vi "Bertta_v04.vi"() -> ()   [LabVIEW 2015]
uses:
  BERTTA.dll
panel:
  in  "Tab Control":T1(tab)
  in  "Description":string
  in  "Project name":string
  in  "User (initials)":string
  out "Mettler":dynamicdata(graph)
  out "?":dynamicdata(graph)
  in  "Balances":bool[](array[boolean])
  out "Waveform Chart 3":dynamicdata(graph)
  out "Table":string[][](table)
  in  "Headers":string[](array[string])
  in  "Seq":dbl[][](array[numeric])=[[20.0, 60.0, 40.0], [60.0, 40.0, 20.0], [100.0, 100.0, 100.0]]
  out "Waveform Chart":dynamicdata(graph)
  in  "PAUSE":bool
  in  "START SEQUENCE":bool
  out "setpoint":dbl
  out "Tcurrent":dbl
  in  "Step":i32
  out "Tinit":dbl
  out "Tset":dbl
  out "Ramp time":dbl
  in  "Heidolph":dbl(slide) scale=0.0..1000.0
  in  "Ismatec":dbl(slide) scale=0.0..160.0
  in  "?":T2(tab)
  out "rc":i32
  in  "Device port":dbl=1.0
  out "Debug msg":dbl
  in  "Device port":dbl=20.0
  in  "Device port":i32=2
  out "Weight":dbl
  out "Weight":dbl
  in  "Device port":i32=6
  in  "Device port":i32=15
  # "1"
  # "2"
  # "3"
  # "4"
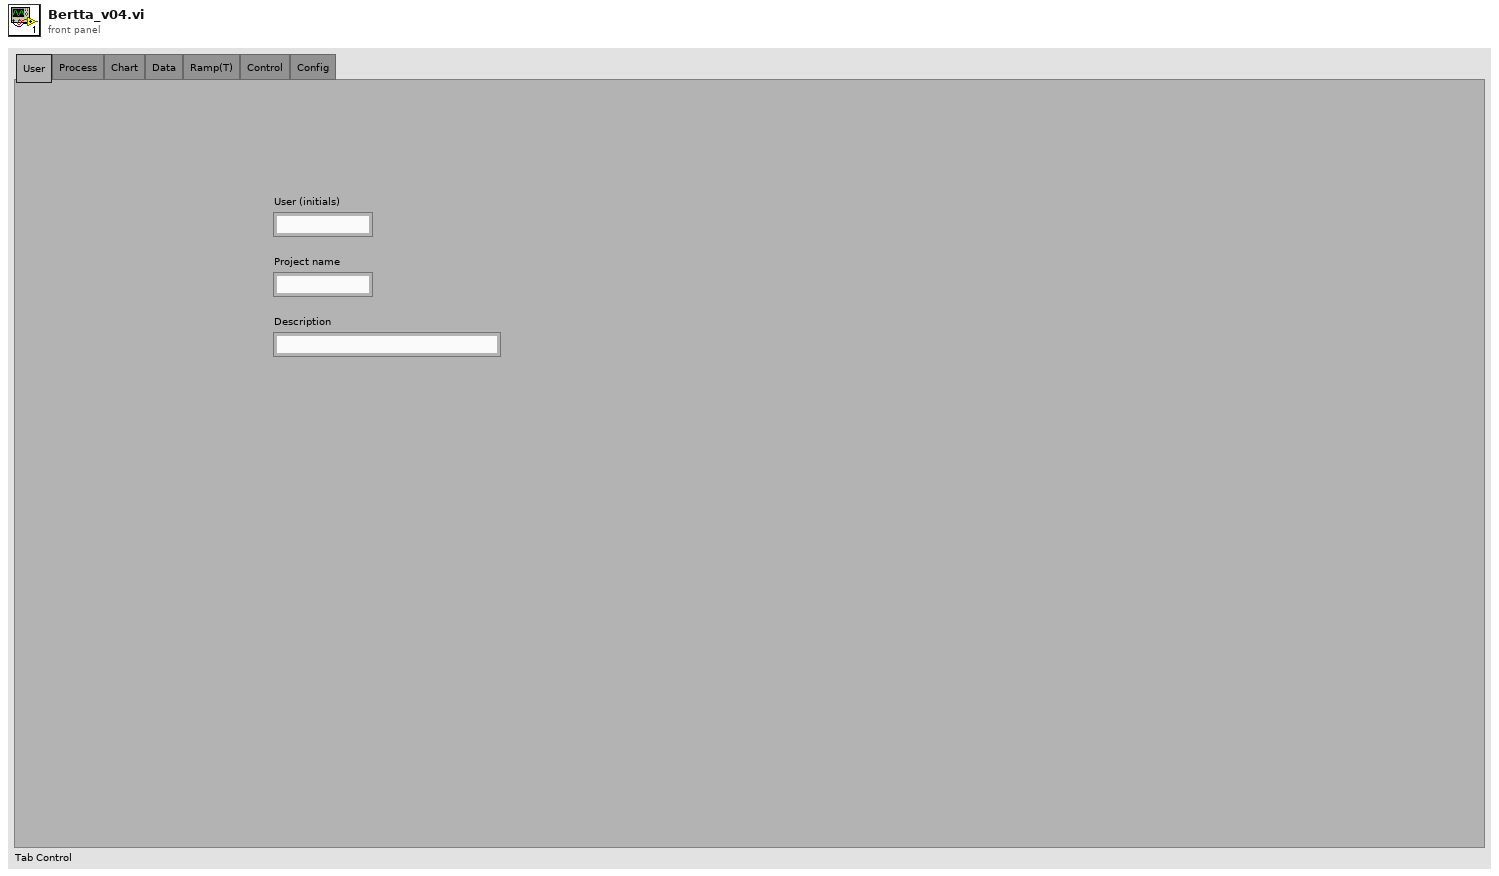
[diagram p1: front panel]
types:
  T1 = enum32{"User", "Process", "Chart", "Data", "Ramp(T)", "Control", "Config"}
  T2 = enum32{"DB / File", "Lauda", "Heidolph", "Mettler 1", "Mettler 2", "Mettler 3", "Ismatec 1"}
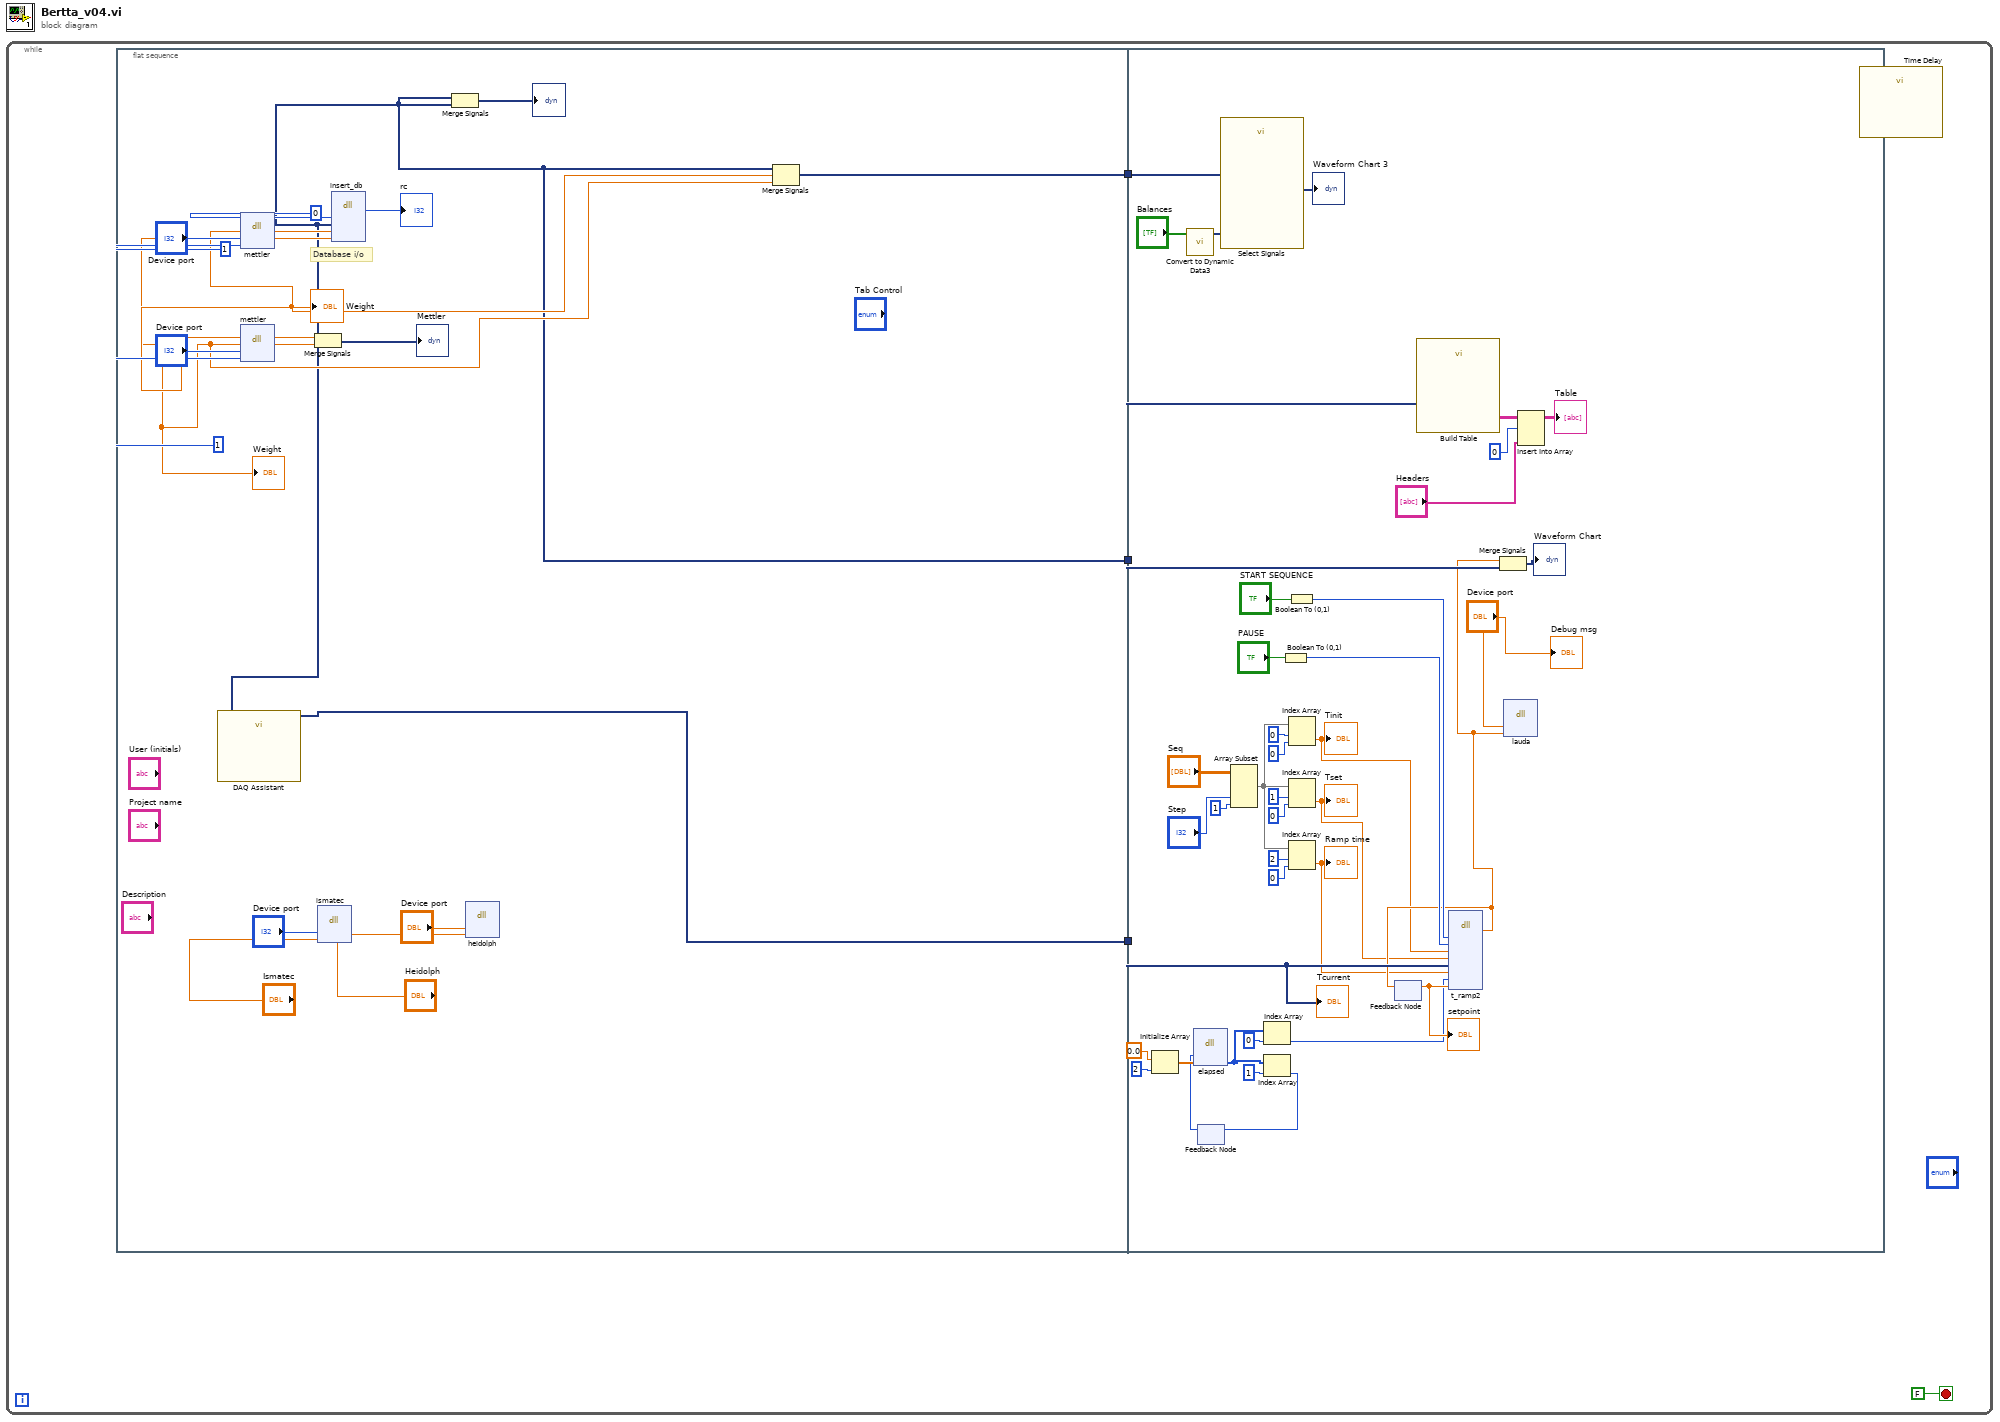
[diagram p0: block diagram]
diagram:
  n1 = while {
    stop <- FALSE stop-if-true
    n2 = flat-sequence {
      tunnel: [w6] -> w3
      tunnel: [w5] -> w2
      tunnel: [w5] -> w1
      tunnel: w3 -> [w53]
      tunnel: w2 -> [w42]
      tunnel: w1 -> [w35]
      frame #0 {
        # "Database i/o"
        n3 = call "DAQ Assistant"() -> ("data"=w5:dynamicdata)  [unwired: 17 in, 2 out]
        n4 = dll-call lib="C:/Users/xlaraser/Documents/Visual Studio 2017/Projects/Bertta/BERTTA/Debug/BERTTA.dll" fn="mettler"("port"="Device port", "msg"=1) -> ("return type"=w8:dbl)  [unwired: 5 in, 2 out]
        "Weight" <- w8
        n5 = dll-call lib="C:/Users/xlaraser/Documents/Visual Studio 2017/Projects/Bertta/BERTTA/Debug/BERTTA.dll" fn="mettler"("port"="Device port", "msg"=1) -> ("return type"=w7:dbl)  [unwired: 5 in, 2 out]
        "Weight" <- w7
        n6 = Merge Signals(w8, w7) -> (→"Mettler":dynamicdata)
        n7 = dll-call lib="C:/Users/xlaraser/Documents/Visual Studio 2017/Projects/Bertta/BERTTA/Debug/BERTTA.dll" fn="ismatec"("port"="Device port", "speed"="Ismatec") -> ()  [unwired: 6 in, 2 out]
        n8 = dll-call lib="C:/Users/xlaraser/Documents/Visual Studio 2017/Projects/Bertta/BERTTA/Debug/BERTTA.dll" fn="insert_db"("heidolph"=0, "lauda"=w5, "mettler1"=w8, "mettler2"=w7) -> ("return type"=→"rc":i32)  [unwired: 7 in, 2 out]
        n9 = Merge Signals(w5, w5) -> (→"?":dynamicdata)
        n10 = dll-call lib="C:/Users/xlaraser/Documents/Visual Studio 2017/Projects/Bertta/BERTTA/Debug/BERTTA.dll" fn="heidolph"("port"="Device port", "speed"="Heidolph") -> ()  [unwired: 6 in, 2 out]
        n11 = Merge Signals(w5, w8, w7) -> (w6:dynamicdata)
      }
      frame #1 {
        n12 = Initialize Array(0.0 ("element"), 2 ("dimension size")) -> (w51:dbl[])
        n13 = call "Convert to Dynamic Data3"("Array"="Balances") -> ("Dynamic Data Type"=w54:dynamicdata)  [unwired: 3 in]
        n14 = feedback #1() -> (w44:i32)  [unwired: 1 in]
        n15 = dll-call lib="C:/Users/xlaraser/Documents/Visual Studio 2017/Projects/Bertta/BERTTA/Debug/BERTTA.dll" fn="elapsed"("last_time"=w44, "params"=w51) -> ("params"=w47:i32[])  [unwired: 5 in, 2 out]
        n16 = call "Select Signals"("Selector Input"=w54, "Signals"=w53) -> ("Signal Out"=→"Waveform Chart 3":dynamicdata)  [unwired: 8 in, 1 out]
        n17 = Array Subset(array="Seq", index (col)="Step", length (col)=1 ("length")) -> (w27:dbl[][])  [unwired: 2 in]
        n18 = Index Array(array=w47, index=0) -> (element=w43:i32)
        n19 = Index Array(array=w47, index=1) -> (element=w45:i32)
        n20 = feedback-in #1(w45) -> ()
        n21 = Boolean To (0,1)(Boolean="PAUSE") -> (0, 1=w39:i16)
        n22 = Boolean To (0,1)(Boolean="START SEQUENCE") -> (0, 1=w40:i16)
        n23 = Index Array(array=w27, index (row)=0, index (col)=0 ("disabled index (col)")) -> (element=w26:dbl)
        "Tinit" <- w26
        n24 = Index Array(array=w27, index (row)=1, index (col)=0 ("disabled index (col)")) -> (element=w22:dbl)
        "Tset" <- w22
        n25 = Index Array(array=w27, index (row)=2, index (col)=0 ("disabled index (col)")) -> (element=w21:dbl)
        "Ramp time" <- w21
        n26 = feedback #2() -> (w52:dbl)  [unwired: 1 in]
        "setpoint" <- w52
        n27 = call "Build Table"("Signals"=w53) -> ("Table"=w57:string[][])  [unwired: 4 in, 6 out]
        n28 = dll-call lib="C:/Users/xlaraser/Documents/Visual Studio 2017/Projects/Bertta/BERTTA/Debug/BERTTA.dll" fn="t_ramp2"("enable"=w40, "pause"=w39, "Tinit"=w26, "Tset"=w22, "Tcurrent"=w42, "ramp_time"=w21, "elapsed"=w43, "sp_old"=w52) -> ("return type"=w34:dbl)  [unwired: 11 in, 2 out]
        n29 = feedback-in #2(w34) -> ()
        n30 = Merge Signals(w34, w35) -> (→"Waveform Chart":dynamicdata)
        n31 = dll-call lib="C:/Users/xlaraser/Documents/Visual Studio 2017/Projects/Bertta/BERTTA/Debug/BERTTA.dll" fn="lauda"("port"="Device port", "set_temp"=w34) -> ()  [unwired: 6 in, 2 out]
        n32 = Insert Into Array(array=w57, index (row)=0, new element="Headers") -> (→"Table":string[][])  [unwired: 1 in]
        "Tcurrent" <- w42
        "Debug msg" <- "Device port"
      }
    }
    n33 = call "Time Delay"() -> ()  [unwired: 11 in, 1 out]
  }
